vi "Read RTU Data.vi"(8 "error in (no error)":errorcluster, 10 "function code":u8=1 format="%x", 11 "HFP Gen in":refnum<class "PL HFP Generator.lvclass">) -> (0 "error out":errorcluster, 2 "data":string, 3 "HFP Gen out":refnum<class "PL HFP Generator.lvclass">)   [LabVIEW 2015, in "PL HFP Generator.lvclass"]
doc: "Reads RTU frame data. Override this VI for not implemented and user-defined Modbus function code(s)."
uses:
  PL HFP Generator.lvclass
  <vilib>/plasmapper/PL Modbus Client/PL Modbus Client.lvclass
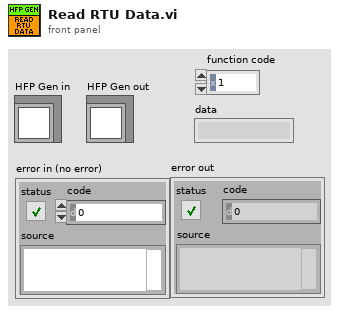
[diagram p1: front panel]
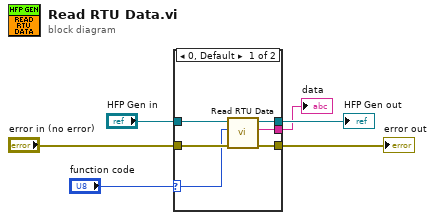
[diagram p0: block diagram]
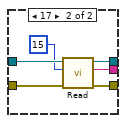
[diagram p2: hidden frame]
diagram:
  n1 = case shown="0, Default" "function code" {
    selector: "function code" -> [w7 _]
    tunnel: "error in (no error)" -> [w8 w18]
    tunnel: [w9 w13] -> w6
    tunnel: "HFP Gen in" -> [w12 w17]
    tunnel: [w11 w14] -> w5
    tunnel: [w10 w15] -> w3
    frame 0, Default {
      n2 = call-parent "Read RTU Data.vi"("error in (no error)"=w8, "function code"=w7, "MODBUS in"=w12) -> ("error out"=w9:errorcluster, "data"=w10:string, "MODBUS out"=w11:refnum<class "PL HFP Generator.lvclass">)  [unwired: 6 in]
    }
    frame 17 {
      n3 = call <vilib>:"Read.vi"("error in (no error)"=w18, "byte count"=u32 15, "MODBUS in"=w17) -> ("error out"=w13:errorcluster, "read buffer"=w15:string, "MODBUS out"=w14:refnum<class "PL HFP Generator.lvclass">)  [unwired: 6 in]
    }
  }
  "HFP Gen out" <- w5
  "data" <- w3
  "error out" <- w6
